vi "Write to Display.vi"(8 "error in (no error)":errorcluster, 11 "Simulated Screen Interface in":refnum<class "Simulated Screen Interface.lvclass">) -> (0 "error out":errorcluster, 3 "Simulated Screen Interface out":refnum<class "Simulated Screen Interface.lvclass">)   [LabVIEW 2017, in "Simulated Screen Interface.lvlib" / "Simulated Screen Interface.lvclass"]
uses:
  Simulated Screen Interface.lvclass
  Screen Interface/Screen Interface/Screen Interface.lvclass
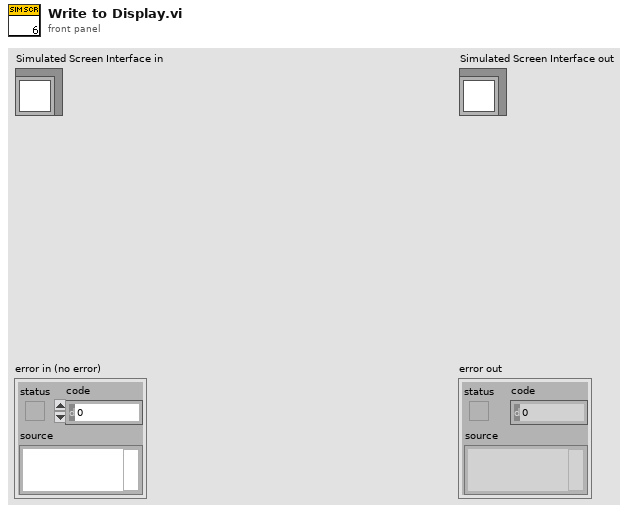
[diagram p1: front panel]
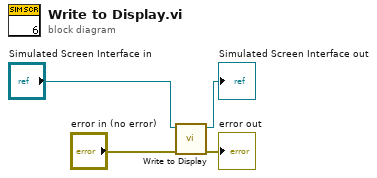
[diagram p0: block diagram]
diagram:
  n1 = call-parent "Write to Display.vi"("error in (no error)"="error in (no error)", "Screen Interface in"="Simulated Screen Interface in") -> ("error out"=→"error out":errorcluster, "Screen Interface out"=→"Simulated Screen Interface out":refnum<class "Simulated Screen Interface.lvclass">)  [unwired: 8 in]
